vi "Quantel Trigger Levels.vi"(10 "New Trigger set":dbl=200.0) -> (2 "Array":dbl[](array[numeric]))   [LabVIEW 2022 SP3]
uses:
  <vilib>/Utility/file.llb/Write To Spreadsheet File (I64).vi
  <vilib>/gmath/NI_Gmath.lvlib
panel:
  out "Quantel array triggers 2":dbl[](array[numeric])
  out "Array 2":dbl[](array[numeric])
  out "Waveform Graph":dbl[](graph)
  in  "Quantel array triggers":dbl[](array[numeric])=[388.0, 422.0, 460.0, 494.0, 532.0, 571.0, 614.0, 652.0, 695.0, 738.0, 781.0, 829.0, 872.0, 920.0, 964.0, 1011.0, 1059.0, 1103.0, 1150.0, 1198.0, 1241.0, 1289.0, 1337.0, 1380.0, 1424.0, 1472.0, 1515.0, 1558.0, 1601.0, 1639.0, 1682.0, 1721.0, 1764.0, 1802.0, 1841.0, 1879.0, 1912.0, 1951.0, 1984.0, 2018.0, 2051.0, 2085.0, 2119.0, 2147.0, 2181.0, 2210.0, 2238.0, 2267.0, 2296.0, 2325.0, 2349.0, 2377.0, 2401.0, 2425.0, 2454.0, 2478.0, 2502.0, 2521.0, 2545.0, 2569.0, 2588.0, 2612.0, 2631.0, 2655.0, 2674.0, 2694.0, 2713.0, 2732.0, 2751.0, 2770.0, 2789.0, 2809.0, 2828.0, 2847.0, 2861.0, 2881.0, 2900.0, 2914.0, 2933.0, 2948.0, 2962.0, 2981.0, 2996.0, 3010.0, 3024.0, 3039.0, 3058.0, 3072.0, 3087.0, 3101.0, 3111.0, 3125.0, 3139.0, 3154.0, 3168.0, 3178.0, 3192.0, 3202.0, 3216.0, 3230.0, 3240.0, 3250.0, 3264.0, 3273.0, 3288.0, 3297.0, 3307.0, 3317.0, 3331.0, 3341.0, 3350.0, 3360.0, 3369.0, 3379.0, 3389.0, 3398.0, 3412.0, 3422.0, 3432.0, 3441.0, 3451.0, 3460.0, 3470.0, 3480.0, 3489.0, 3504.0, 3513.0, 3523.0, 3532.0, 3547.0, 3556.0, 3566.0, 3580.0, 3590.0, 3604.0, 3614.0, 3628.0, 3643.0, 3652.0, 3666.0, 3681.0, 3695.0, 3710.0, 3724.0, 3738.0, 3753.0, 3772.0, 3786.0, 3805.0, 3820.0, 3839.0, 3858.0, 3877.0, 3897.0, 3916.0, 3935.0, 3954.0, 3978.0, 3997.0, 4021.0, 4045.0, 4069.0, 4093.0, 4117.0, 4141.0, 4165.0, 4194.0, 4218.0, 4246.0, 4275.0, 4304.0, 4333.0, 4361.0, 4395.0, 4424.0, 4457.0, 4491.0, 4524.0, 4558.0, 4591.0, 4630.0, 4663.0, 4702.0, 4740.0, 4778.0, 4821.0, 4860.0, 4903.0, 4946.0, 4989.0, 5032.0, 5080.0, 5128.0, 5176.0, 5224.0, 5277.0, 5329.0, 5382.0, 5435.0, 5488.0, 5545.0, 5603.0, 5665.0, 5722.0, 5785.0, 5847.0, 5914.0, 5976.0, 6044.0, 6115.0, 6183.0, 6254.0, 6326.0, 6403.0, 6480.0, 6556.0, 6633.0, 6710.0, 6791.0, 6873.0, 6959.0, 7040.0, 7127.0, 7213.0, 7299.0, 7390.0, 7476.0, 7568.0, 7659.0, 7750.0, 7841.0, 7932.0, 8023.0, 8114.0, 8210.0, 8301.0, 8392.0, 8483.0, 8574.0, 8660.0, 8751.0, 8838.0, 8924.0, 9010.0, 9096.0, 9178.0, 9259.0, 9336.0, 9413.0, 9489.0, 9561.0, 9628.0, 9700.0, 9762.0, 9825.0, 9887.0]
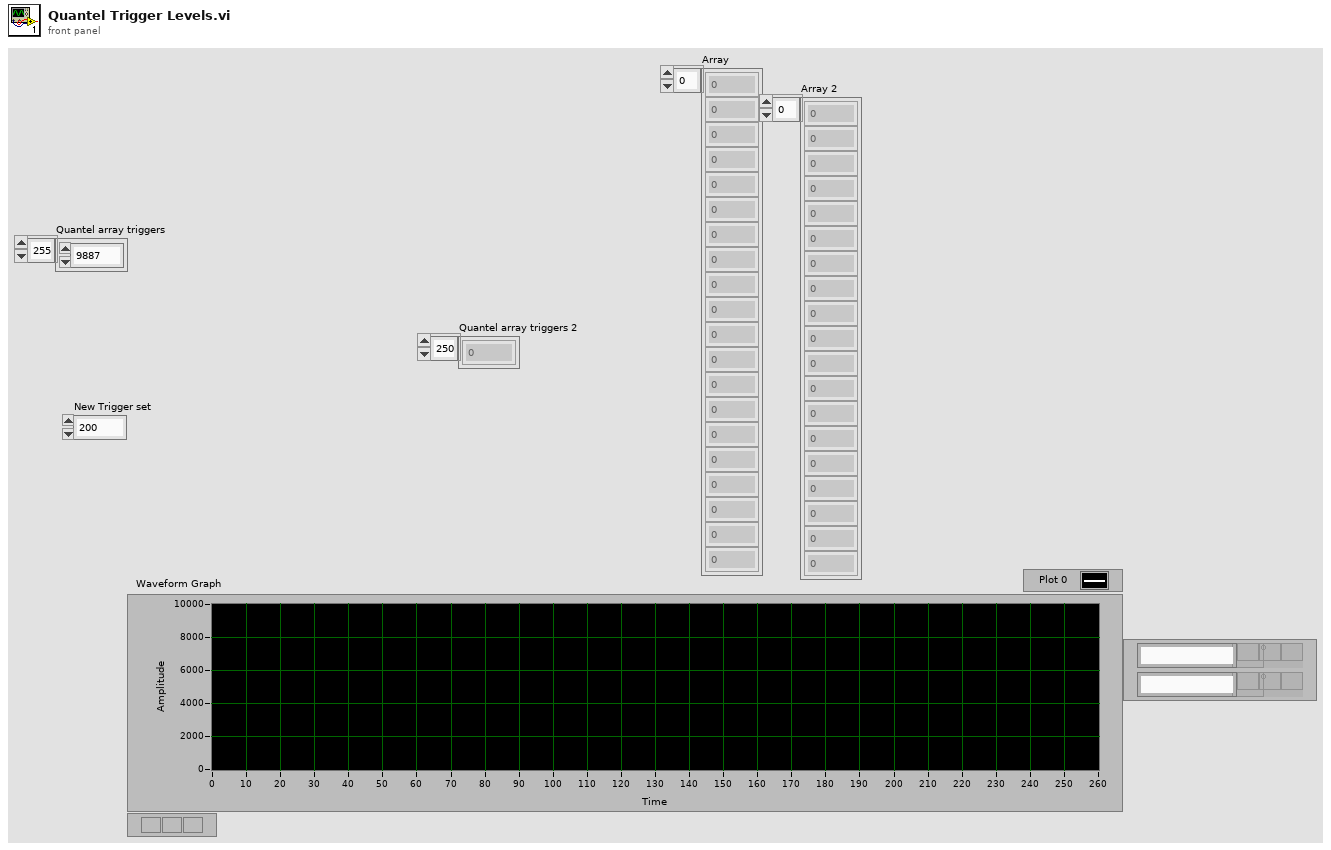
[diagram p1: front panel]
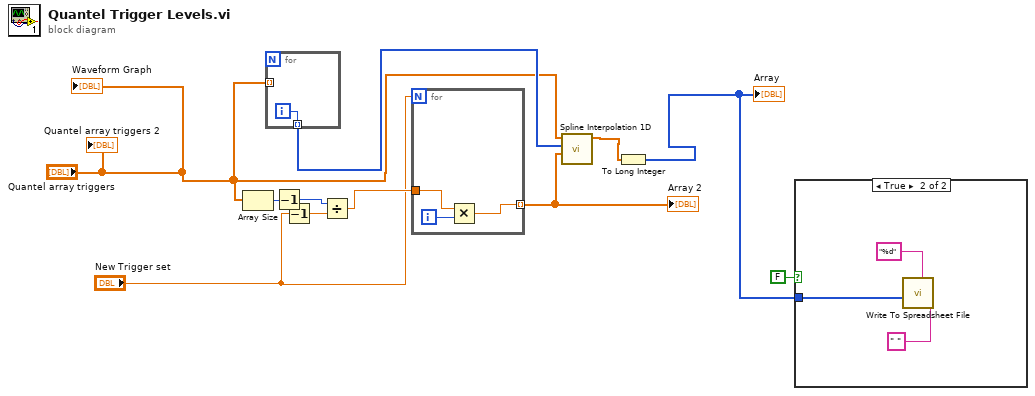
[diagram p0: block diagram]
diagram:
  n1 = Array Size(array="Quantel array triggers") -> (size(s)=w11:i32)
  n2 = for {
    tunnel: "Quantel array triggers" -> [_] mode=indexing
    tunnel: [w12] -> w7 mode=indexing
    i -> [w12]
  }
  n3 = Decrement(x=w11) -> (x-1=w6:i32)
  n4 = Decrement(x="New Trigger set") -> (x-1=w5:dbl)
  n5 = Divide(x=w6, y=w5) -> (x/y=w10:dbl)
  n6 = for {
    N: "New Trigger set" -> [_]
    tunnel: w10 -> [w14]
    tunnel: [w13] -> w8 mode=indexing
    i -> [w15]
    n7 = Multiply(x=w14, y=w15) -> (x*y=w13:dbl)
  }
  "Array 2" <- w8
  n8 = call <vilib>:"Spline Interpolation 1D.vi"("xi"=w8, "X"=w7, "Y"="Quantel array triggers") -> ("yi"=w4:dbl[])  [unwired: 6 in, 2 out]
  n9 = To Long Integer(number=w4) -> (32bit integer=w3:i32[])
  "Array" <- w3
  n10 = case shown="True" FALSE {
    tunnel: w3 -> [_ w18]
    frame False {
    }
    frame True {
      n11 = call-poly <vilib>:"Write To Spreadsheet File.vi"("delimiter (\\t)"=" " ("delimiter (\\t)"), "format (%d)"="%d", "1D data"=w18) -> ()  [unwired: 5 in, 1 out]
    }
  }
  "Waveform Graph" <- "Quantel array triggers"
  "Quantel array triggers 2" <- "Quantel array triggers"
